vi "MT EbN0 Calculation(PAM).vi"(0 "Recieved waveform":T3={"t0"=0.0, "dt"=1.0, "Y"=[]} {"Y" format="%.3f"; "dt" format="%^.2e"; "t0" format="%.4f"}, 1 "pulse shaping filter coefficients":dbl[](array[numeric]) format="%.2f", 5 "PAM system parameters":T1={"samples per symbol (16)"=16, "symbol map"=[]} {"symbol map" format="%.3f"}, 7 "synchronization parameters":T2 {"sync sequence" format="%.2f"}, 9 "matched filter coefficients":dbl[](array[numeric]) format="%.2f", 11 "error in (no error)":errorcluster, 12 "reset? (T)":bool=TRUE) -> (4 "Eb/N0":dbl, 6 "Eb/N0(dB)":dbl, 15 "error out":errorcluster)   [LabVIEW 2020, in "niDMT.lvlib"]
uses:
  <vilib>/addons/Modulation/niDMT.lvlib
  <vilib>/addons/Modulation/Analog/controls/Complex Data Waveform.ctl
  <vilib>/Analysis/2dsp.llb/1D Convolution (DBL).vi
  <vilib>/Analysis/NI_AALPro.lvlib
  <vilib>/addons/Modulation/niAMT.lvlib
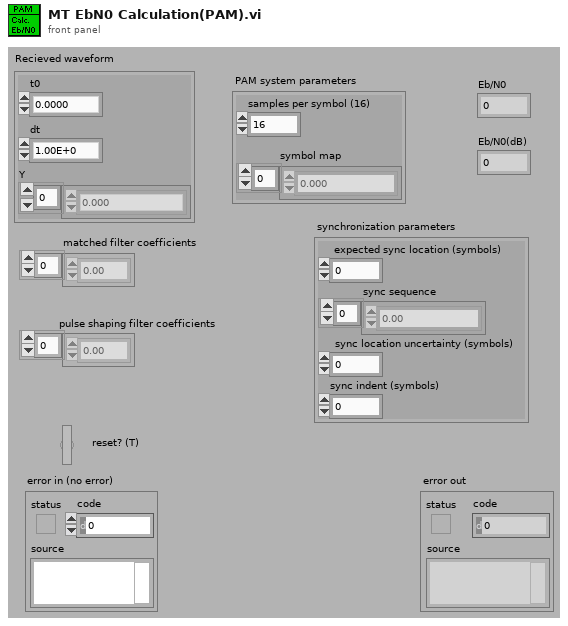
[diagram p1: front panel]
types:
  T1 = cluster{"samples per symbol (16)":i32, "symbol map":cdb[]}
  T2 = cluster{"expected sync location (symbols)":i32, "sync sequence":cdb[], "sync location uncertainty (symbols)":i32, "sync indent (symbols)":i32}
  T3 = typedef "niAMT.lvlib/Complex Data Waveform.ctl" = cluster{"t0":dbl, "dt":dbl, "Y":cdb[]}
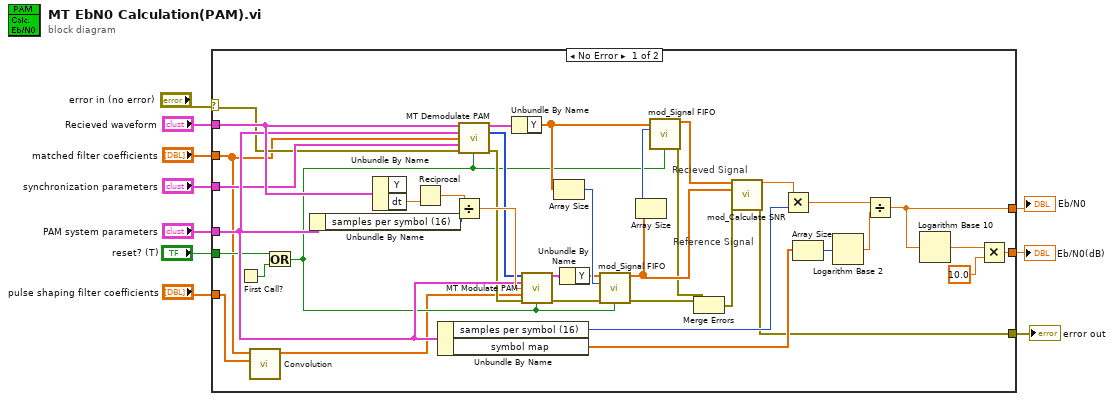
[diagram p0: block diagram]
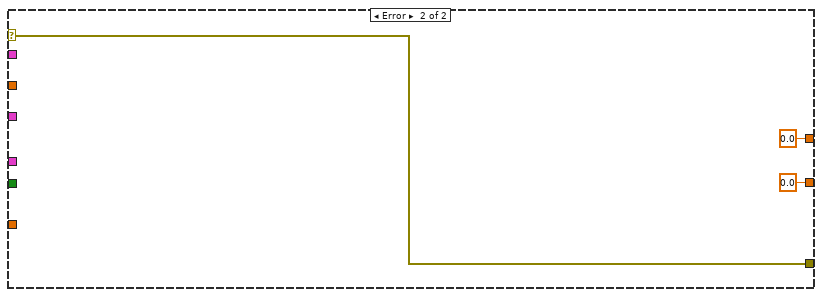
[diagram p2: hidden frame]
diagram:
  n1 = case shown="No Error" "error in (no error)" {
    selector: "error in (no error)" -> [w18 w50]
    tunnel: "matched filter coefficients" -> [w14 _]
    tunnel: "pulse shaping filter coefficients" -> [w13 _]
    tunnel: [w31 0.0] -> w8
    tunnel: [w28 0.0] -> w7
    tunnel: "Recieved waveform" -> [w27 _]
    tunnel: "PAM system parameters" -> [w26 _]
    tunnel: "synchronization parameters" -> [w25 _]
    tunnel: [w19 w50] -> w3
    tunnel: "reset? (T)" -> [w17 _]
    frame No Error {
      # "Recieved Signal"
      # "Reference Signal"
      n2 = First Call?() -> (First Call?: T/F=w16:bool)
      n3 = call-poly <vilib>:"Convolution.vi"("Y"=w13, "X"=w14) -> ("X * Y"=w12:dbl[])  [unwired: 1 in, 8 out]
      n4 = Or(x=w17, y=w16) -> (x .or. y?=w15:bool)
      n5 = Unbundle By Name(w26) -> ("samples per symbol (16)"=w47:i32)
      n6 = Unbundle By Name(w27) -> ("dt"=w49:dbl)  [unwired: 1 out]
      n7 = Reciprocal(x=w49) -> (1/x=w44:dbl)
      n8 = Unbundle By Name(w26) -> ("samples per symbol (16)"=w45:i32, "symbol map"=w43:cdb[])
      n9 = Divide(x=w44, y=w47) -> (x/y=w48:dbl)
      n10 = call <vilib>:"MT Demodulate PAM.vi"("input complex waveform"=w27, "PAM system parameters"=w26, "matched filter coefficients"=w14, "synchronization parameters"=w25, "error in (no error)"=w18, "reset? (T)"=w15) -> ("recovered complex waveform"=w11:T3, "output bit stream"=w41:i8[], "error out"=w24:errorcluster)  [unwired: 1 in, 6 out]
      n11 = Unbundle By Name(w11) -> ("Y"=w37:cdb[])
      n12 = call <vilib>:"MT Modulate PAM.vi"("input bit stream"=w41, "PAM system parameters"=w26, "symbol rate (Hz)"=w48, "pulse shaping filter coefficients"=w12, "error in (no error)"=w24, "reset? (T)"=w15) -> ("output complex waveform"=w39:T3, "error out"=w23:errorcluster)  [unwired: 1 in, 7 out]
      n13 = Array Size(array=w37) -> (size(s)=w36:i32)
      n14 = Unbundle By Name(w39) -> ("Y"=w35:cdb[])
      n15 = call <vilib>:"mod_Signal FIFO.vi"("Signal In"=w35, "Output Length"=w36, "error in (no error)"=w23, "Reset? (T)"=w15) -> ("Signal Out"=w34:cdb[], "error out"=w22:errorcluster)  [unwired: 10 out]
      n16 = Array Size(array=w34) -> (size(s)=w33:i32)
      n17 = call <vilib>:"mod_Signal FIFO.vi"("Signal In"=w37, "Output Length"=w33, "Reset? (T)"=w15) -> ("Signal Out"=w38:cdb[], "error out"=w21:errorcluster)  [unwired: 1 in, 10 out]
      n18 = Merge Errors(w21, w22) -> (w20:errorcluster)
      n19 = call <vilib>:"mod_Calculate SNR.vi"("Recieved Waveform"=w38, "Reference Waveform"=w34, "error in (no error)"=w20) -> ("SNR"=w46:dbl, "error out"=w19:errorcluster)  [unwired: 11 out]
      n20 = Multiply(x=w46, y=w45) -> (x*y=w40:dbl)
      n21 = Array Size(array=w43) -> (size(s)=w42:i32)
      n22 = Logarithm Base 2(1:w42) -> (0:w32:dbl)
      n23 = Divide(x=w40, y=w32) -> (x/y=w31:dbl)
      n24 = Logarithm Base 10(1:w31) -> (0:w30:dbl)
      n25 = Multiply(x=w30, y=10.0) -> (x*y=w28:dbl)
    }
    frame Error {
    }
  }
  "Eb/N0" <- w8
  "Eb/N0(dB)" <- w7
  "error out" <- w3
